vi "FGSD Calibration tool ver 1.1.2.vi"() -> ()   [LabVIEW 2018]
uses:
  <vilib>/Utility/NIReport.llb/NI_report.lvclass
  <vilib>/Utility/NIReport.llb/Excel/NI_Excel.lvclass
  <vilib>/Utility/NIReport.llb/Report Type.ctl
  <vilib>/DAQmx/read.llb/DAQmx Read (Analog Wfm 1Chan NSamp).vi
  <vilib>/Utility/NIReport.llb/Append Text Table to Report (wrap).vi
  <vilib>/DAQmx/create/channels.llb/DAQmx Create Channel (AI-Voltage-Basic).vi
  <vilib>/DAQmx/configure/timing.llb/DAQmx Timing (Sample Clock).vi
  <vilib>/DAQmx/miscellaneous.llb/DAQmx Fill In Error Info.vi
  <vilib>/Utility/NIReport.llb/Append Numeric Table to Report (wrap).vi
  <vilib>/Utility/NIReport.llb/NI_ReportGenerationCore.lvlib
  <resource>/objmgr/daqmx.rc
panel:
  in  "Run Next":bool
  in  "Continue":bool
  in  "Unit":enum16{"oz.in", "lbf-ft.", "lbf-in.", "N-m"}(ring)
  in  "Sensor ID:":tag
  in  "samples per channel":i32=4000
  in  "rate":dbl=500.0 format="%#_13g"
  in  "milliseconds to wait":u32=1000
  out "Cycles":i32=10
  out "Average":dbl[](array[numeric])=[2.9362440950071025]
  out "Template":refnum<class "NI_report.lvclass">
  out "Upper Limit":dbl=2.12
  out "Lower Limit":dbl=1.88
  out "output array":dbl[][](array[numeric])=[[3.9379769276696557, 2.0, 2.0, 3.7231645789771317, 3.939138075500426], [2.0, 2.0, 3.7939945966541258, 3.968166771269686, 2.0]]
  in  "stop":bool
  out "Torque":dbl=3.9379769276696557 format="%0.2f"
  out "Waveform Graph 2":waveform(dbl)(graph)={"t0"=timestamp(3654803301.2825823 s since 1904-01-01), "dt"=0.000333325, "Y"=array[6000 elements], "attributes"=variant("NI_ChannelName"=variant(string "6003/ai0"), "NI_UnitDescription"=variant(string "oz.in"))}
  out "Torque:":dbl=2.0
  in  "Humidity(%):":string="40"
  in  "Temp(F):":string="75"
  in  "FG Serial Number:":string="0211932-0056"
  in  "User Name:":string="Kyle Watts"
  in  "FG Model:":string(combo)="FG-40i"
  in  "Cal Dir:":string(combo)="CW"
  # "FGSD Calibration Tester ver1.1.2"
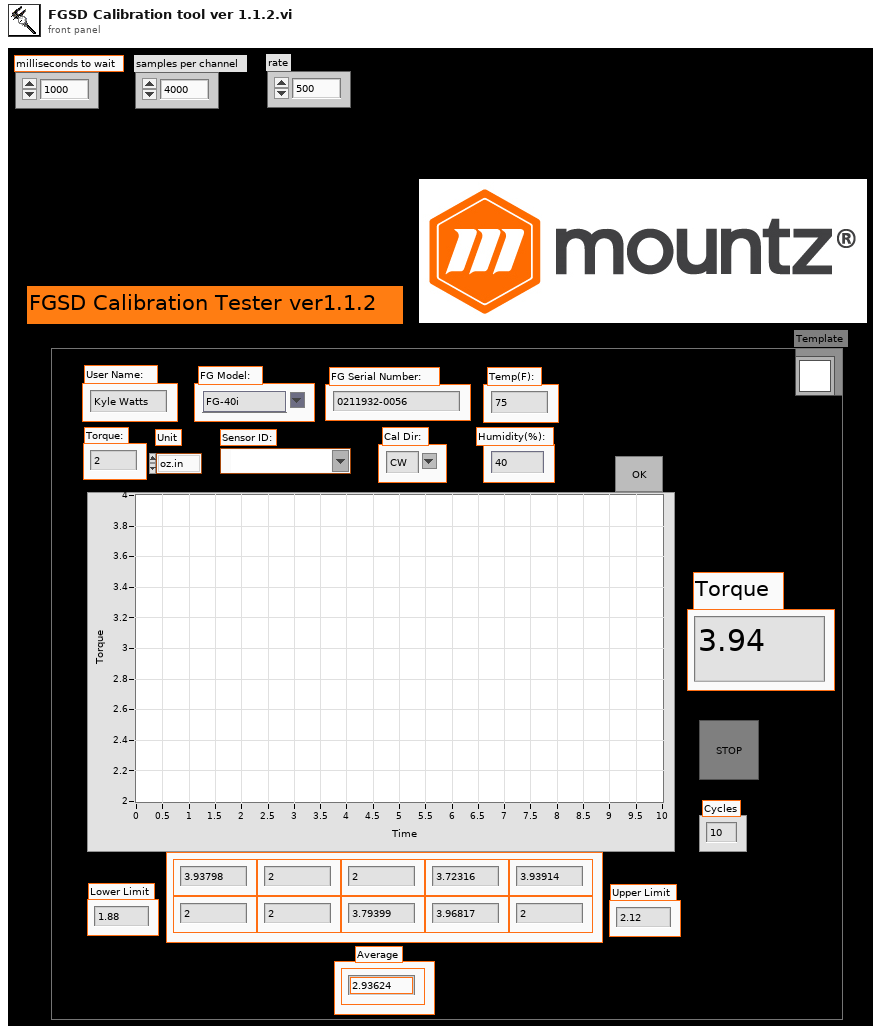
[diagram p1: front panel]
types:
  T1 = enum16{"Initialize ", "Set Torque", "Read Torque"}
  T2 = enum16{"Initialize ", "Set Torque", "Read Torque", "Save data"}
  T3 = cluster{"position (excel)":cluster{"row":i32, "column":i32}, "name (excel)":string, "bookmark (word)":string}
  T4 = cluster{"Charset (-1)":i16, "Weight (-1)":i16, "Name":string, "Size":string}
  T5 = typedef "NI_ReportGenerationCore.lvlib/Report Type.ctl" = enum16{"HTML", "Word", "Excel"}
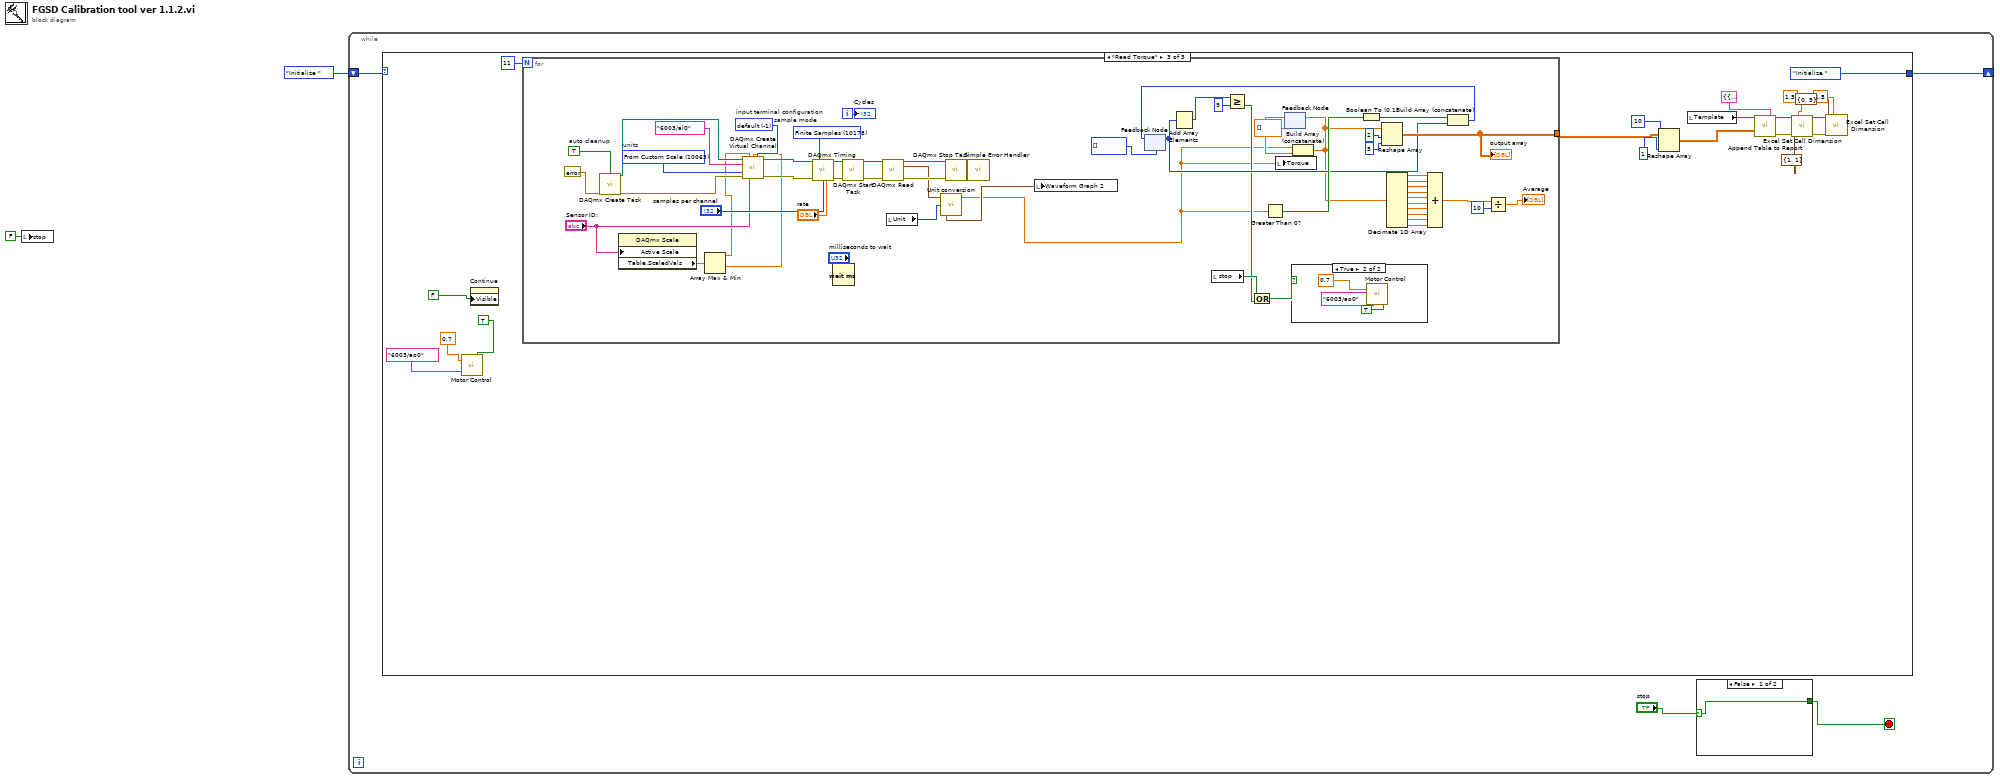
[diagram p0: block diagram]
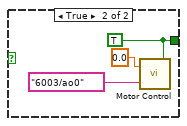
[diagram p2: hidden frame]
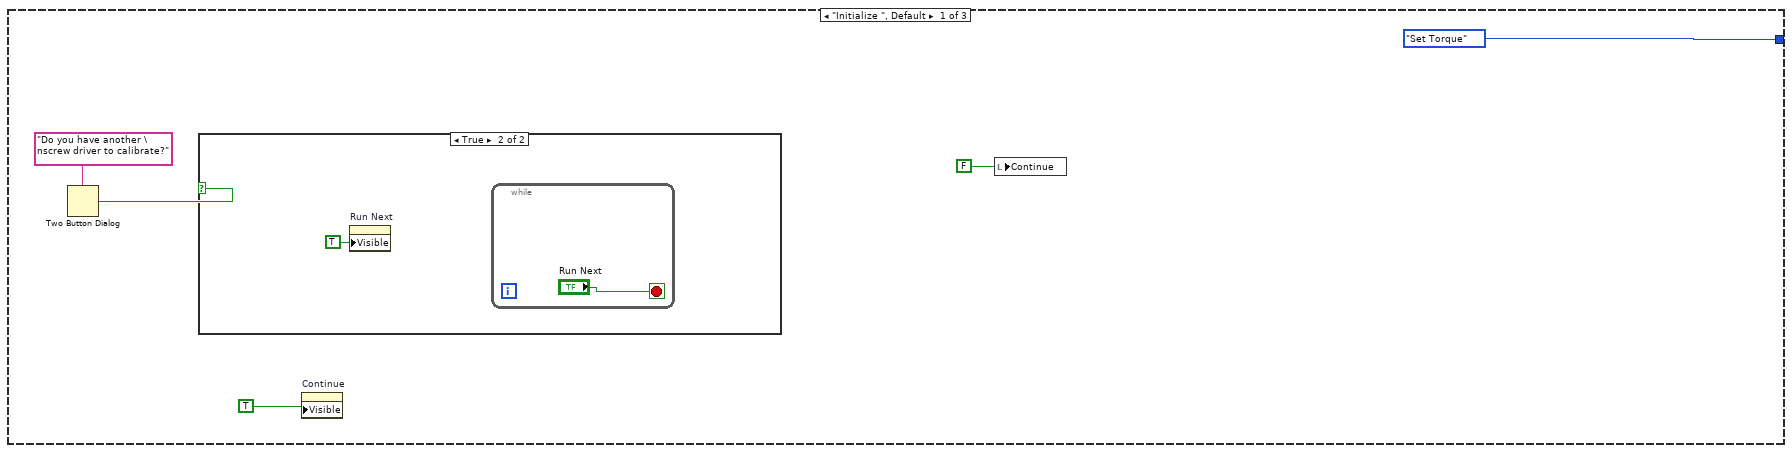
[diagram p3: hidden frame]
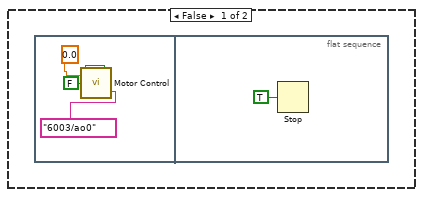
[diagram p4: hidden frame]
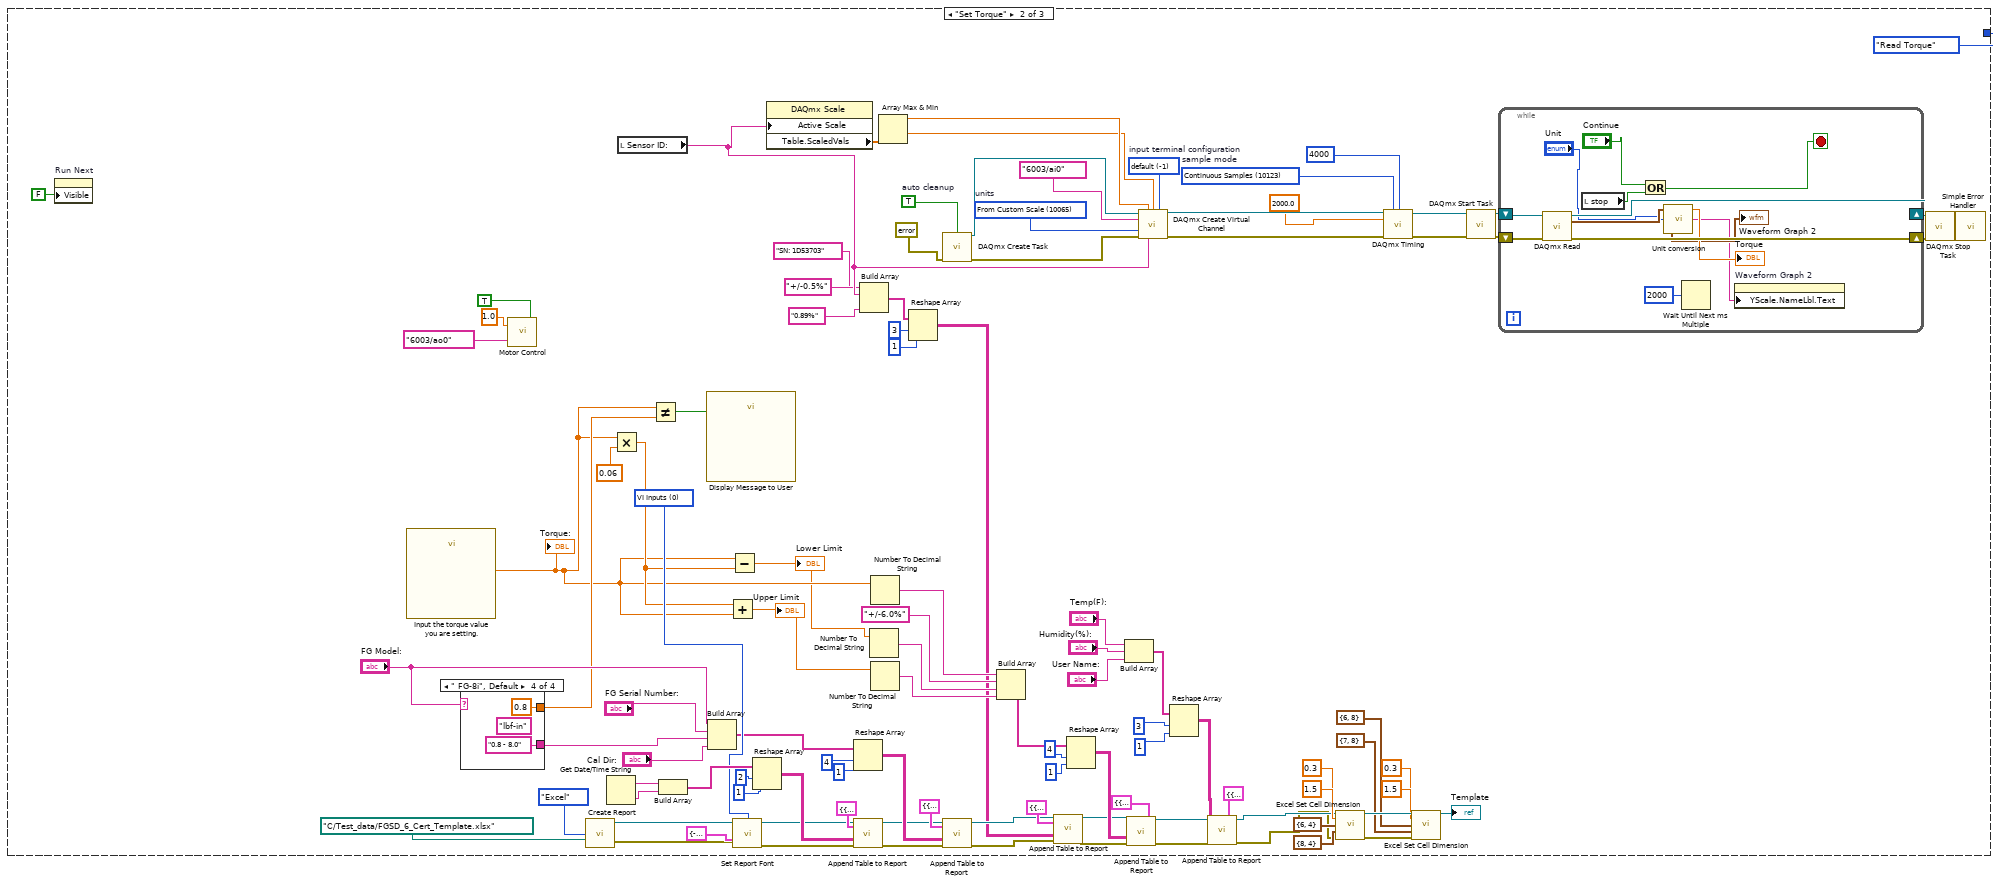
[diagram p5: hidden frame]
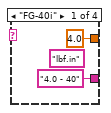
[diagram p6: hidden frame]
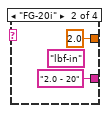
[diagram p7: hidden frame]
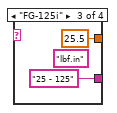
[diagram p8: hidden frame]
diagram:
  n1 = local write "stop"(FALSE ("stop")) -> ()
  n2 = while {
    shift-right: [w5] -> _
    shift-left: T1."Initialize " -> [w6]
    stop <- w3 stop-if-true
    n3 = case shown="\"Read Torque\"" w6 {
      tunnel: [T2."Set Torque" T2."Read Torque" T2."Initialize "] -> w5
      frame "Initialize ", Default {
        n4 = Two Button Dialog(message="Do you have another \nscrew driver to calibrate?") -> (T button?=w12:bool)  [unwired: 2 in]
        n5 = case shown="True" w12 {
          frame False {
            n6 = flat-sequence {
              frame #0 {
                n7 = call "Motor Control.vi"("Run"=FALSE, "physical channels"=tag "6003/ao0", "Speed"=0.0) -> ()
              }
              frame #1 {
                n8 = Stop(stop? (T)=TRUE) -> ()
              }
            }
          }
          frame True {
            n9 = property on="Run Next" class="Bool"("Visible"=TRUE) -> ()  [unwired: 2 in, 2 out]
            n10 = while {
              stop <- "Run Next" stop-if-true
            }
          }
        }
        n11 = property on="Continue" class="Bool (strict)"("Visible"=TRUE) -> ()  [unwired: 2 in, 2 out]
        n12 = local write "Continue"(FALSE ("Continue")) -> ()
      }
      frame "Set Torque" {
        w69 = 10123 items=["Finite Samples"=10178, "Continuous Samples"=10123, "Hardware Timed Single Point"=12522]  # sample mode
        w67 = -1 items=["default"=-1, "RSE"=10083, "NRSE"=10078, "Differential"=10106, "Pseudodifferential"=12529]  # input terminal configuration
        w66 = 10065 items=["Volts"=10348, "From Custom Scale"=10065]  # units
        w63 = TRUE  # auto cleanup
        w111 = u16 0 items=["VI Inputs", "Font Dialog Box"] ("font settings source (VI Inputs)")
        n13 = property on="Run Next" class="Bool"("Visible"=FALSE) -> ()  [unwired: 2 in, 2 out]
        n14 = call "Input the torque value you are setting."() -> ("Torque"=w45:dbl)  [unwired: 17 in, 2 out]
        "Torque:" <- w45
        n15 = case shown="\" FG-8i\", Default" "FG Model:" {
          tunnel: ["4.0 - 40" "2.0 - 20" "25 - 125" "0.8 - 8.0"] -> w48
          tunnel: [4.0 2.0 25.5 0.8] -> w82
          frame "FG-40i" {
            (unwired) "lbf.in"
          }
          frame "FG-20i" {
            (unwired) "lbf-in"
          }
          frame "FG-125i" {
            (unwired) "lbf.in"
          }
          frame " FG-8i", Default {
            (unwired) "lbf-in"
          }
        }
        n16 = call "Motor Control.vi"("Run"=TRUE, "physical channels"=tag "6003/ao0", "Speed"=1.0) -> ()
        n17 = call <vilib>:"Create Report.vi"("report type"=Report_Type."Excel", "template (empty)"=path "C:/Test_data/FGSD_6_Cert_Template.xlsx") -> ("report out"=w110:refnum<class "NI_report.lvclass">, "error out"=w109:errorcluster)  [unwired: 12 in]
        n18 = Get Date/Time String() -> (date string=w116:string, time string=w117:string)  [unwired: 3 in]
        n19 = Multiply(x=w45, y=0.06) -> (x*y=w78:dbl)
        n20 = local read "Sensor ID:"() -> (w38:tag)
        n21 = Not Equal?(x=w45, y=w82) -> (x != y?=w81:bool)
        n22 = Build Array(w116, w117) -> (w120:string[])
        n23 = call "Display Message to User"("Enable"=w81) -> ()  [unwired: 9 in, 2 out]
        n24 = Build Array("FG Model:", "FG Serial Number:", w48, "Cal Dir:") -> (w94:string[])
        n25 = Add(x=w78, y=w45) -> (x+y=w39:dbl)
        "Upper Limit" <- w39
        n26 = Subtract(x=w45, y=w78) -> (x-y=w40:dbl)
        "Lower Limit" <- w40
        n27 = call-dynamic "Set Report Font.vi"("report in"=w110, "font settings source (VI Inputs)"=w111, "font settings"=T4 {"Charset (-1)"=-1, "Weight (-1)"=-1, "Name"="Calibri", "Size"=" 14"}, "error in (no error)"=w109) -> ("report out"=w107:refnum<class "NI_report.lvclass">, "error out"=w108:errorcluster)  [unwired: 9 in, 1 out]
        n28 = Reshape Array(w120, 2 ("dimension size"), 1 ("dimension size")) -> (w119:string[][])
        n29 = property class="DAQmx Scale"("Active Scale"=w38) -> ("Table.ScaledVals"=w53:dbl[])  [unwired: 2 in, 2 out]
        n30 = Reshape Array(w94, 4 ("dimension size"), 1 ("dimension size")) -> (w93:string[][])
        n31 = call-poly <vilib>:"Append Table to Report.vi"("report in"=w107, "MS Office parameters"=T3 {"position (excel)"={"row"=1, "column"=11}, "name (excel)"="", "bookmark (word)"=""}, "text data"=w119, "error in (no error)"=w108) -> ("report out"=w91:refnum<class "NI_report.lvclass">, "error out"=w90:errorcluster)  [unwired: 8 in, 2 out]
        n32 = Build Array("SN: 1D53703", w38, "+/-0.5%", "0.89%") -> (w35:string[])
        n33 = Number To Decimal String(number=w40) -> (decimal integer string=w42:string)  [unwired: 1 in]
        n34 = Number To Decimal String(number=w45) -> (decimal integer string=w44:string)  [unwired: 1 in]
        n35 = Number To Decimal String(number=w39) -> (decimal integer string=w41:string)  [unwired: 1 in]
        n36 = Array Max & Min(array=w53) -> (max value=w52:dbl, min value=w51:dbl)  [unwired: 2 out]
        n37 = Reshape Array(w35, 3 ("dimension size"), 1 ("dimension size")) -> (w32:string[][])
        n38 = call <vilib>:"DAQmx Create Task.vi"("auto cleanup"=w63, "error in"=errorcluster {"status"=FALSE, "code"=0, "source"=""}) -> ("task out"=w64:refnum<k21>, "error out"=w62:errorcluster)  [unwired: 12 in]
        n39 = call-poly <vilib>:"Append Table to Report.vi"("report in"=w91, "MS Office parameters"=T3 {"position (excel)"={"row"=11, "column"=1}, "name (excel)"="", "bookmark (word)"=""}, "text data"=w93, "error in (no error)"=w90) -> ("report out"=w113:refnum<class "NI_report.lvclass">, "error out"=w114:errorcluster)  [unwired: 8 in, 2 out]
        n40 = Build Array(w44, "+/-6.0%", w42, w41) -> (w89:string[])
        n41 = call-poly <vilib>:"Append Table to Report.vi"("report in"=w113, "MS Office parameters"=T3 {"position (excel)"={"row"=16, "column"=5}, "name (excel)"="", "bookmark (word)"=""}, "text data"=w32, "error in (no error)"=w114) -> ("report out"=w27:refnum<class "NI_report.lvclass">, "error out"=w46:errorcluster)  [unwired: 8 in, 2 out]
        n42 = Reshape Array(w89, 4 ("dimension size"), 1 ("dimension size")) -> (w86:string[][])
        n43 = Build Array("Temp(F):", "Humidity(%):", "User Name:") -> (w83:string[])
        n44 = call-poly <vilib>:"Append Table to Report.vi"("report in"=w27, "MS Office parameters"=T3 {"position (excel)"={"row"=16, "column"=1}, "name (excel)"="", "bookmark (word)"=""}, "text data"=w86, "error in (no error)"=w46) -> ("report out"=w25:refnum<class "NI_report.lvclass">, "error out"=w26:errorcluster)  [unwired: 8 in, 2 out]
        n45 = call-poly <vilib>:"DAQmx Create Virtual Channel.vi"("task in"=w64, "maximum value"=w52, "minimum value"=w51, "input terminal configuration"=w67, "physical channels"=tag "6003/ai0", "units"=w66, "error in"=w62, "custom scale name"=w38) -> ("task out"=w68:refnum<k21>, "error out"=w65:errorcluster)  [unwired: 6 in]
        n46 = Reshape Array(w83, 3 ("dimension size"), 1 ("dimension size")) -> (w28:string[][])
        n47 = call-poly <vilib>:"Append Table to Report.vi"("report in"=w25, "MS Office parameters"=T3 {"position (excel)"={"row"=12, "column"=5}, "name (excel)"="", "bookmark (word)"=""}, "text data"=w28, "error in (no error)"=w26) -> ("report out"=w24:refnum<class "NI_report.lvclass">, "error out"=w23:errorcluster)  [unwired: 8 in, 2 out]
        n48 = call <vilib>:"Excel Set Cell Dimension.vi"("report in"=w24, "width (-1)"=1.5, "height (-1)"=0.3, "start (-1, -1)"=cluster{"row":i32, "column":i32} {"row"=6, "column"=4}, "end (-1, -1)"=cluster{"row":i32, "column":i32} {"row"=8, "column"=4}, "error in (no error)"=w23) -> ("report out"=w102:refnum<class "NI_report.lvclass">, "error out"=w101:errorcluster)  [unwired: 8 in]
        n49 = call-poly <vilib>:"DAQmx Timing.vi"("task/channels in"=w68, "sample mode"=w69, "samples per channel"=4000, "rate"=2000.0, "error in"=w65) -> ("task out"=w71:refnum<k21>, "error out"=w60:errorcluster)  [unwired: 9 in]
        n50 = call <vilib>:"Excel Set Cell Dimension.vi"("report in"=w102, "width (-1)"=1.5, "height (-1)"=0.3, "start (-1, -1)"=cluster{"row":i32, "column":i32} {"row"=6, "column"=8}, "end (-1, -1)"=cluster{"row":i32, "column":i32} {"row"=7, "column"=8}, "error in (no error)"=w101) -> ("report out"=→"Template":refnum<class "NI_report.lvclass">)  [unwired: 8 in, 1 out]
        n51 = call <vilib>:"DAQmx Start Task.vi"("task/channels in"=w71, "error in"=w60) -> ("task out"=w73:refnum<k21>, "error out"=w72:errorcluster)  [unwired: 12 in]
        n52 = while {
          shift-right: [w137] -> w58
          shift-left: w73 -> [w139]
          shift-right: [w136] -> w57
          shift-left: w72 -> [w138]
          stop <- w134 stop-if-true
          n53 = call-poly <vilib>:"DAQmx Read.vi"("task/channels in"=w139, "error in"=w138) -> ("task out"=w137:refnum<k21>, "data"=w132:waveform(dbl), "error out"=w136:errorcluster)  [unwired: 11 in]
          n54 = local read "stop"() -> (w135:bool)
          n55 = Or(x="Continue", y=w135) -> (x .or. y?=w134:bool)
          n56 = call "Unit conversion.vi"("Convert to"="Unit", "data in"=w132) -> ("Unit"=w128:string, "Torque"=→"Torque":dbl, "waveform out"=→"Waveform Graph 2":waveform(dbl))  [unwired: 1 in]
          n57 = Wait Until Next ms Multiple(millisecond multiple=u32 2000) -> ()  [unwired: 1 out]
          n58 = property on="Waveform Graph 2" class="WFGraph (strict)"("YScale.NameLbl.Text"=w128) -> ()  [unwired: 2 in, 2 out]
        }
        n59 = call <vilib>:"DAQmx Stop Task.vi"("task/channels in"=w58, "error in"=w57) -> ("error out"=w56:errorcluster)  [unwired: 12 in, 1 out]
        n60 = call <vilib>:"Simple Error Handler.vi"("error in (no error)"=w56) -> ()  [unwired: 4 in, 5 out]
      }
      frame "Read Torque" {
        n61 = call "Motor Control.vi"("Run"=TRUE, "physical channels"=tag "6003/ao0", "Speed"=0.7) -> ()
        n62 = property on="Continue" class="Bool (strict)"("Visible"=FALSE) -> ()  [unwired: 2 in, 2 out]
        n63 = for {
          N: 11 -> [_]
          tunnel: [w225] -> w164
          i -> [w199]
          w184 = 10178 items=["Finite Samples"=10178, "Continuous Samples"=10123, "Hardware Timed Single Point"=12522]  # sample mode
          w181 = -1 items=["default"=-1, "RSE"=10083, "NRSE"=10078, "Differential"=10106, "Pseudodifferential"=12529]  # input terminal configuration
          w179 = 10065 items=["Volts"=10348, "From Custom Scale"=10065]  # units
          w178 = TRUE  # auto cleanup
          n64 = call <vilib>:"DAQmx Create Task.vi"("auto cleanup"=w178, "error in"=errorcluster {"status"=FALSE, "code"=0, "source"=""}) -> ("task out"=w190:refnum<k21>, "error out"=w189:errorcluster)  [unwired: 12 in]
          n65 = property class="DAQmx Scale"("Active Scale"="Sensor ID:") -> ("Table.ScaledVals"=w174:dbl[])  [unwired: 2 in, 2 out]
          n66 = Array Max & Min(array=w174) -> (max value=w173:dbl, min value=w172:dbl)  [unwired: 2 out]
          n67 = call-poly <vilib>:"DAQmx Create Virtual Channel.vi"("task in"=w190, "maximum value"=w173, "minimum value"=w172, "input terminal configuration"=w181, "physical channels"=tag "6003/ai0", "units"=w179, "error in"=w189, "custom scale name"="Sensor ID:") -> ("task out"=w192:refnum<k21>, "error out"=w191:errorcluster)  [unwired: 6 in]
          n68 = call-poly <vilib>:"DAQmx Timing.vi"("task/channels in"=w192, "sample mode"=w184, "samples per channel"="samples per channel", "rate"="rate", "error in"=w191) -> ("task out"=w193:refnum<k21>, "error out"=w188:errorcluster)  [unwired: 9 in]
          n69 = Wait (ms)(milliseconds to wait="milliseconds to wait") -> ()  [unwired: 1 out]
          n70 = call <vilib>:"DAQmx Start Task.vi"("task/channels in"=w193, "error in"=w188) -> ("task out"=w195:refnum<k21>, "error out"=w194:errorcluster)  [unwired: 12 in]
          n71 = call-poly <vilib>:"DAQmx Read.vi"("task/channels in"=w195, "error in"=w194) -> ("task out"=w187:refnum<k21>, "data"=w171:waveform(dbl), "error out"=w186:errorcluster)  [unwired: 11 in]
          n72 = local read "Unit"() -> (w168:enum16{"oz.in", "lbf-ft.", "lbf-in.", "N-m"})
          n73 = call "Unit conversion.vi"("Convert to"=w168, "data in"=w171) -> ("Torque"=w169:dbl, "waveform out"=w170:waveform(dbl))  [unwired: 1 in, 1 out]
          n74 = call <vilib>:"DAQmx Stop Task.vi"("task/channels in"=w187, "error in"=w186) -> ("error out"=w185:errorcluster)  [unwired: 12 in, 1 out]
          n75 = call <vilib>:"Simple Error Handler.vi"("error in (no error)"=w185) -> ()  [unwired: 4 in, 5 out]
          n76 = local write "Waveform Graph 2"(w170) -> ()
          n77 = feedback #1(i16[] []) -> (w220:i16[])
          n78 = Add Array Elements(numeric array=w220) -> (sum=w222:i16)
          n79 = local read "stop"() -> (w200:bool)
          n80 = Greater Or Equal?(x=w222, y=i16 9) -> (x >= y?=w176:bool)
          n81 = Or(x=w200, y=w176) -> (x .or. y?=w198:bool)
          n82 = Greater Than 0?(x=w169) -> (x > 0?=w224:bool)
          n83 = local write "Torque"(w169) -> ()
          n84 = feedback #2(dbl[] []) -> (w217:dbl[])
          n85 = case shown="True" w198 {
            frame False {
            }
            frame True {
              n86 = call "Motor Control.vi"("Run"=TRUE, "physical channels"=tag "6003/ao0", "Speed"=0.7) -> ()
            }
          }
          n87 = Build Array (concatenate)(w169, w217) -> (w213:dbl[])
          n88 = feedback-in #2(w213) -> ()
          n89 = Boolean To (0,1)(Boolean=w224) -> (0, 1=w223:i16)
          n90 = Reshape Array(w213, 2 ("dimension size"), 5 ("dimension size")) -> (w225:dbl[][])
          "output array" <- w225
          n91 = Decimate 1D Array(w213) -> (w212:dbl[], w211:dbl[], w210:dbl[], w209:dbl[], w208:dbl[], w207:dbl[], w206:dbl[], w205:dbl[], w204:dbl[], w203:dbl[])
          n92 = Compound Arithmetic op=ADD(w212, w211, w210, w209, w208, w207, w206, w205, w204, w203) -> (w197:dbl[])
          n93 = Build Array (concatenate)(w223, w220) -> (w221:i16[])
          n94 = feedback-in #1(w221) -> ()
          n95 = Divide(x=w197, y=10) -> (x/y=→"Average":dbl[])
          "Cycles" <- w199
        }
        n96 = Reshape Array(w164, 10 ("dimension size"), 1 ("dimension size")) -> (w163:dbl[][])
        n97 = local read "Template"() -> (w161:refnum<class "NI_report.lvclass">)
        n98 = call-poly <vilib>:"Append Table to Report.vi"("report in"=w161, "MS Office parameters"=T3 {"position (excel)"={"row"=23, "column"=1}, "name (excel)"="", "bookmark (word)"=""}, "numerical data"=w163) -> ("report out"=w155:refnum<class "NI_report.lvclass">, "error out"=w152:errorcluster)  [unwired: 9 in, 2 out]
        n99 = call <vilib>:"Excel Set Cell Dimension.vi"("report in"=w155, "width (-1)"=1.5 ("column width (1)"), "start (-1, -1)"=cluster{"row":i32, "column":i32} {"row"=1, "column"=1}, "error in (no error)"=w152) -> ("report out"=w154:refnum<class "NI_report.lvclass">, "error out"=w153:errorcluster)  [unwired: 10 in]
        n100 = call <vilib>:"Excel Set Cell Dimension.vi"("report in"=w154, "width (-1)"=1.5, "end (-1, -1)"=cluster{"row":i32, "column":i32} {"row"=0, "column"=5}, "error in (no error)"=w153) -> ()  [unwired: 10 in, 2 out]
      }
    }
    n101 = case shown="False" "stop" {
      selector: "stop" -> [w7 _]
      tunnel: [w7 w8] -> w3
      frame False {
      }
      frame True {
        w8 = TRUE ("Run")
        n102 = call "Motor Control.vi"("Run"=w8, "physical channels"=tag "6003/ao0", "Speed"=0.0) -> ()
      }
    }
  }
